vi "updateBP.vi"(8 "error in (no error)":errorcluster, 11 "reference in":refnum<class "Devices Controller.lvclass">) -> (0 "error out":errorcluster, 3 "reference out":refnum<class "Devices Controller.lvclass">)   [LabVIEW 2014, in "Devices Controller.lvclass"]
uses:
  Devices Controller.lvclass
  deviceType.ctl
  APP/bodpod_class/bodpod.lvclass
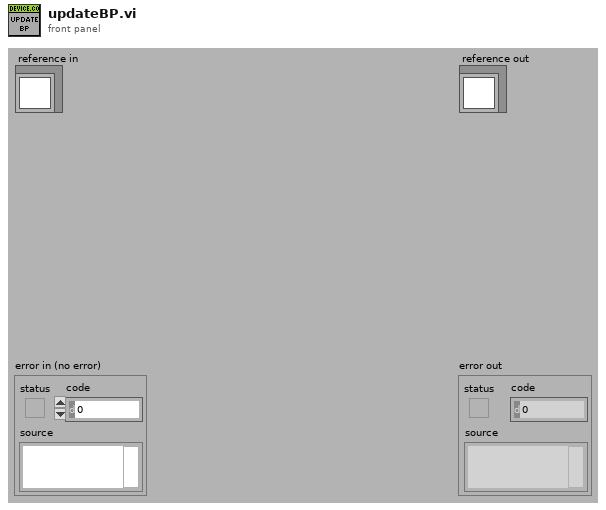
[diagram p1: front panel]
types:
  T1 = typedef "Devices Controller.lvclass/deviceType.ctl" = enum16{"k5", "k4b2", "fitmate", "cpet", "rmr", "bodyBoxPft", "bp", "pp"}
  T2 = cluster{"deviceType":T1, "S/N":string, "SW":string, "Description":string, "Account":string, "System's Location":string, "End User":string, "Email":string, "City":string, "FollowUp Sent":string, "FollowUp Accepted":string, "Note":string}
  T3 = typedef "Devices Controller.lvclass/ObjectAttributesRef.ctl" = refnum<data-value>
  T4 = typedef "Devices Controller.lvclass/ObjectAttributes.ctl" = cluster{"MyAttribute":dbl, "file_controller_ref":refnum<class "File Controller.lvclass">, "data":string[][][], "devices_refs":cluster{"k4b2_refs":refnum<class "k4b2.lvclass">[], "rmr_refs":refnum<class "rmr.lvclass">[], "bod_pod_refs":refnum<class "bodpod.lvclass">[], "cpet_refs":refnum<class "cpet.lvclass">[], "fitmate_refs":refnum<class "fitmate.lvclass">[], "pea_pod_refs":refnum<class "peapod.lvclass">[], "k5_refs":refnum<class "k5.lvclass">[], "bb-pft_refs":refnum<class "bb-pft.lvclass">[]}}
  T5 = cluster{"data[0]":string, "data[1]":string, "data[2]":string, "data[3]":string, "data[4]":string, "data[5]":string, "data[6]":string, "data[7]":string, "data[8]":string}
  T6 = cluster{"[0]":string, "[1]":string, "[2]":string, "[3]":string, "[4]":string, "[5]":string, "[6]":string, "[7]":string, "[8]":string}
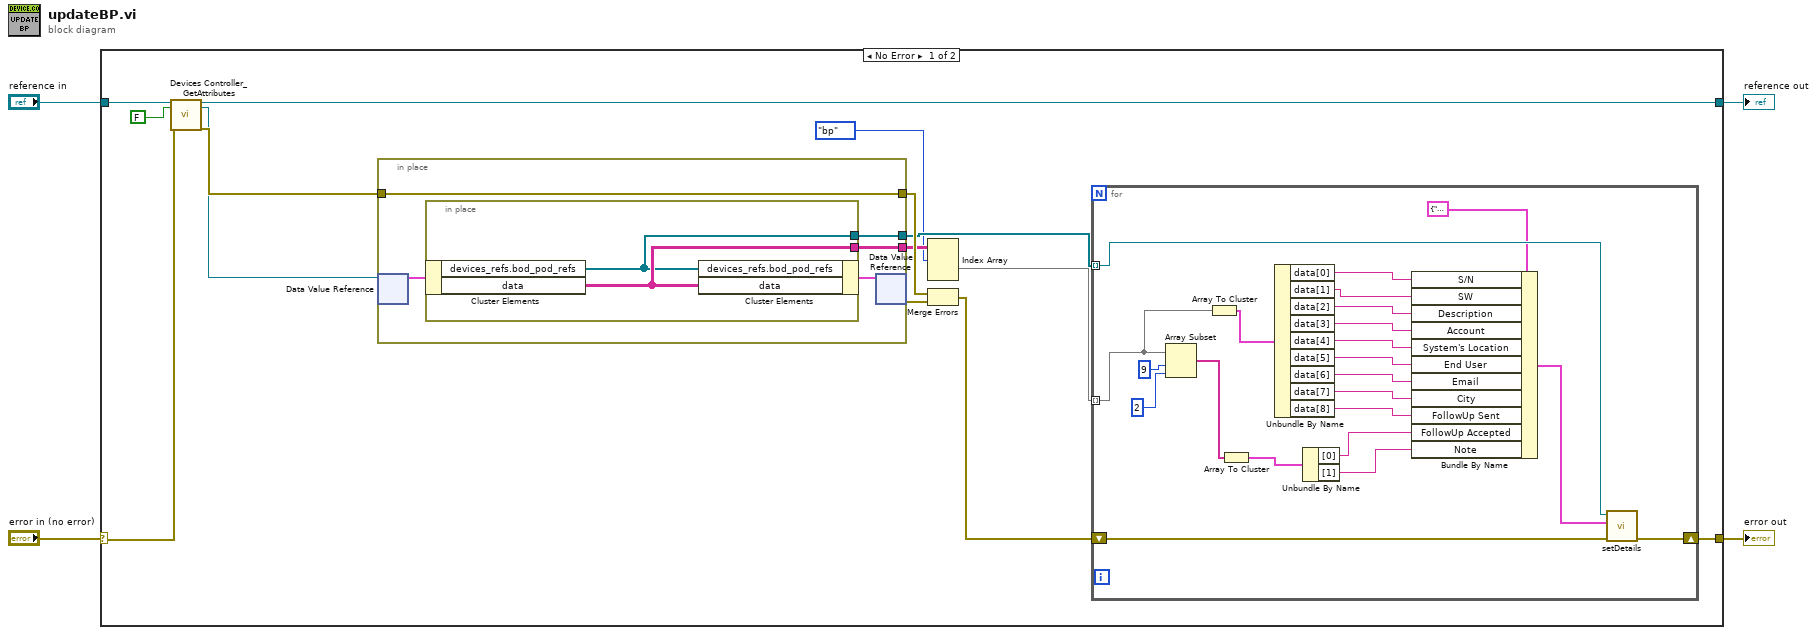
[diagram p0: block diagram]
diagram:
  n1 = case shown="No Error" "error in (no error)" {
    selector: "error in (no error)" -> [w14 w49]
    tunnel: [w9 w49] -> w3
    tunnel: [w12 w48] -> w1
    tunnel: "reference in" -> [w16 w48]
    frame No Error {
      n2 = call "Devices Controller_GetAttributes.vi"("reference in"=w16, "return data? (T)"=FALSE, "error in (no error)"=w14) -> ("reference out"=w12:refnum<class "Devices Controller.lvclass">, "attributes ref"=w11:T3, "error out"=w13:errorcluster)  [unwired: 13 in, 1 out]
      n3 = in-place {
        in-place-border: w13 -> [w43]
        in-place-border: [w43] -> w17
        in-place-border: [w42] -> w7
        in-place-border: [w41] -> w8
        n4 = in-place-dvr #1(w11) -> (w44:T4)  [unwired: 1 out]
        n5 = in-place {
          in-place-border: [w47] -> w42
          in-place-border: [w46] -> w41
          n6 = in-place-cluster #2(w44) -> ("devices_refs.bod_pod_refs"=w46:refnum<class "bodpod.lvclass">[], "data"=w47:string[][][])
          n7 = in-place-cluster #2("devices_refs.bod_pod_refs"=w46, "data"=w47) -> (w45:T4)
        }
        n8 = in-place-dvr #1(w45) -> (w18:errorcluster)  [unwired: 1 out]
      }
      n9 = Index Array(array=w7, index (dim 0)=deviceType."bp" ("deviceType")) -> (element=w6:string[][])  [unwired: 2 in]
      n10 = Merge Errors(w17, w18) -> (w10:errorcluster)
      n11 = for {
        tunnel: w8 -> [w38] mode=indexing
        tunnel: w6 -> [w32] mode=indexing
        shift-right: [w39] -> w9
        shift-left: w10 -> [w40]
        n12 = Array Subset(array=w32, index=9, length=2) -> (w34:string[])
        n13 = Array To Cluster(array=w32) -> (cluster=w37:T5)
        n14 = Array To Cluster(array=w34) -> (cluster=w33:T6)
        n15 = Unbundle By Name(w37) -> ("data[0]"=w31:string, "data[1]"=w30:string, "data[2]"=w29:string, "data[3]"=w28:string, "data[4]"=w27:string, "data[5]"=w26:string, "data[6]"=w25:string, "data[7]"=w24:string, "data[8]"=w23:string)
        n16 = Unbundle By Name(w33) -> ("[0]"=w22:string, "[1]"=w19:string)
        n17 = Bundle By Name(cluster=T2 {"deviceType"=enum."k5", "S/N"="", "SW"="", "Description"="", "Account"="", "System's Location"="", "End User"="", "Email"="", "City"="", "FollowUp Sent"="", "FollowUp Accepted"="", "Note"=""} ("details"), "S/N"=w31, "SW"=w30, "Description"=w29, "Account"=w28, "System's Location"=w27, "End User"=w26, "Email"=w25, "City"=w24, "FollowUp Sent"=w23, "FollowUp Accepted"=w22, "Note"=w19) -> (w20:T2)
        n18 = call "setDetails.vi"("error in (no error)"=w40, "details"=w20, "reference in"=w38) -> ("error out"=w39:errorcluster)  [unwired: 7 in, 1 out]
      }
    }
    frame Error {
    }
  }
  "error out" <- w3
  "reference out" <- w1
